vi "Maps-Set Center.vi"(0 "Google Maps Resource Out in":T1, 7 "Center Position":cluster{"Latitude":string, "Longitude":string}, 11 "error in (no error)":errorcluster) -> (4 "Google Maps Resource Out out":T1, 15 "error out":errorcluster)   [LabVIEW 2020]
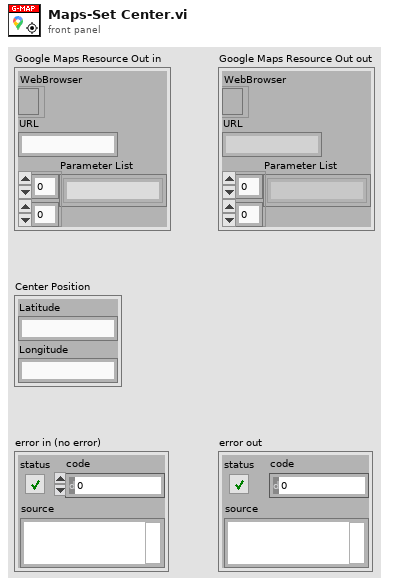
[diagram p1: front panel]
types:
  T1 = cluster{"WebBrowser":refnum<k7>, "URL":string, "Parameter List":string[][]}
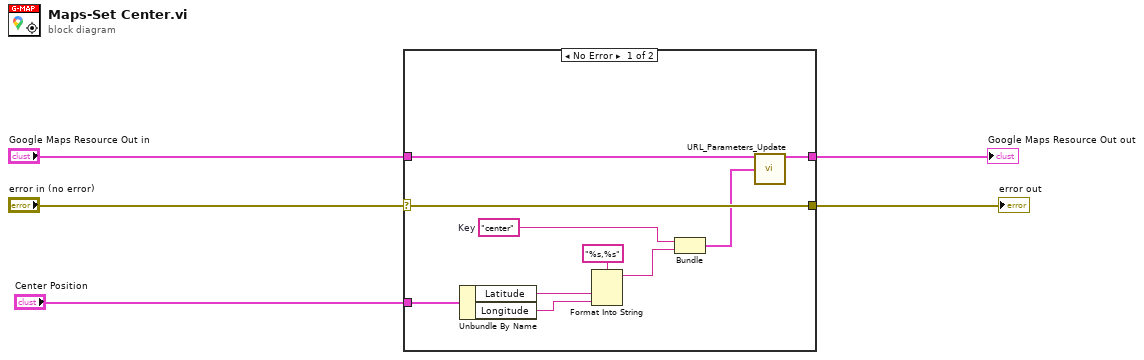
[diagram p0: block diagram]
diagram:
  n1 = case shown="No Error" "error in (no error)" {
    selector: "error in (no error)" -> [w15 w16]
    tunnel: "Google Maps Resource Out in" -> [w8 w17]
    tunnel: [w6 w17] -> w2
    tunnel: [w15 w16] -> w4
    tunnel: "Center Position" -> [w14 _]
    frame No Error {
      w10 = "center"  # Key
      n2 = Unbundle By Name(w14) -> ("Latitude"=w13:string, "Longitude"=w12:string)
      n3 = Format Into String(format string="%s,%s", w13, w12) -> (resulting string=w9:string)  [unwired: 2 in, 1 out]
      n4 = Bundle("Key"=w10, w9) -> (w7:cluster{"Key":string, string})  [unwired: 1 in]
      n5 = call "URL_Parameters_Update.vi"("Google Maps Resource In"=w8, "URL Parameter"=w7) -> ("Google Maps Resource Out"=w6:T1)  [unwired: 13 in]
    }
    frame Error {
    }
  }
  "error out" <- w4
  "Google Maps Resource Out out" <- w2
